vi "TxBfrPkt - Add Channels.vi"(6 "Ext Buffer?":bool, 7 "Add Port Channel?":bool, 8 "error in (no error)":errorcluster, 11 "Node Ptr":T1 format="%.0x") -> (0 "error out":errorcluster, 3 "Node Ptr out":T1 format="%.0x")   [LabVIEW 2016, in "UDP-Custom-Device System Explorer.lvlib"]
uses:
  UDP-Custom-Device System Explorer.lvlib
  <vilib>/NI Veristand/Custom Device API/Custom Device Item Ref.ctl
  <vilib>/NI Veristand/Custom Device API/Custom Device Channel.ctl
  <vilib>/NI Veristand/Custom Device API/Custom Device Channel Type.ctl
  <vilib>/NI VeriStand/Custom Device API/Custom Device API.lvlib
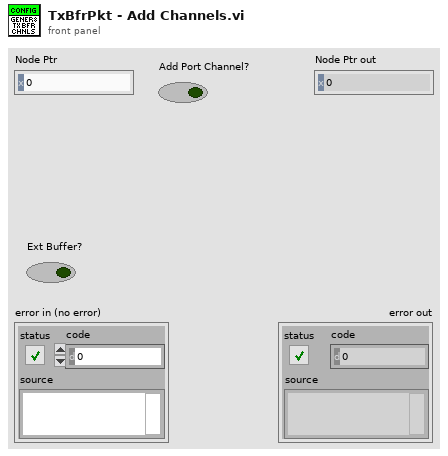
[diagram p1: front panel]
types:
  T1 = typedef "Custom Device API.lvlib/Custom Device Item Ref.ctl" = u64
  T2 = typedef "Custom Device API.lvlib/Custom Device Channel.ctl" = cluster{"Type":T3, "Units":string, "Default Value":dbl, "Faultable":bool, "Scalable":bool}
  T3 = typedef "Custom Device API.lvlib/Custom Device Channel Type.ctl" = enum16{"Input", "Output"}
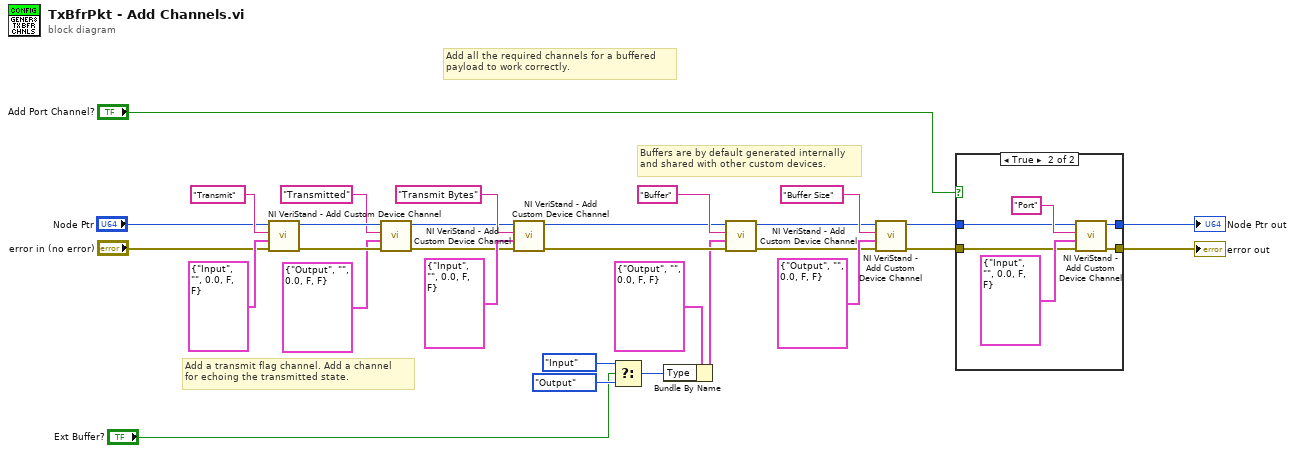
[diagram p0: block diagram]
diagram:
  # "Add a transmit flag channel. Add a channel\nfor echoing the transmitted state."
  # "Buffers are by default generated internally\nand shared with other custom devices."
  # "Add all the required channels for a buffered\npayload to work correctly."
  n1 = call <vilib>:"NI VeriStand - Add Custom Device Channel.vi"("error in (no error)"="error in (no error)", "Channel"=T2 {"Type"=enum."Input", "Units"="", "Default Value"=0.0, "Faultable"=FALSE, "Scalable"=FALSE}, "Channel Name"="Transmit", "Parent Ref in"="Node Ptr") -> ("error out"=w15:errorcluster, "Parent Ref out"=w17:T1)  [unwired: 4 in, 2 out]
  n2 = call <vilib>:"NI VeriStand - Add Custom Device Channel.vi"("error in (no error)"=w15, "Channel"=T2 {"Type"=enum."Output", "Units"="", "Default Value"=0.0, "Faultable"=FALSE, "Scalable"=FALSE}, "Channel Name"="Transmitted", "Parent Ref in"=w17) -> ("error out"=w14:errorcluster, "Parent Ref out"=w16:T1)  [unwired: 4 in, 2 out]
  n3 = call <vilib>:"NI VeriStand - Add Custom Device Channel.vi"("error in (no error)"=w14, "Channel"=T2 {"Type"=enum."Input", "Units"="", "Default Value"=0.0, "Faultable"=FALSE, "Scalable"=FALSE}, "Channel Name"="Transmit Bytes", "Parent Ref in"=w16) -> ("error out"=w24:errorcluster, "Parent Ref out"=w25:T1)  [unwired: 4 in, 2 out]
  n4 = Select(t=Custom_Device_Channel_Type."Input" ("Type"), s="Ext Buffer?", f=Custom_Device_Channel_Type."Output" ("Type")) -> (s? t:f=w21:T3)
  n5 = Bundle By Name(cluster=T2 {"Type"=enum."Output", "Units"="", "Default Value"=0.0, "Faultable"=FALSE, "Scalable"=FALSE} ("Channel"), "Type"=w21) -> (w18:T2)
  n6 = call <vilib>:"NI VeriStand - Add Custom Device Channel.vi"("error in (no error)"=w24, "Channel"=w18, "Channel Name"="Buffer", "Parent Ref in"=w25) -> ("error out"=w8:errorcluster, "Parent Ref out"=w9:T1)  [unwired: 4 in, 2 out]
  n7 = call <vilib>:"NI VeriStand - Add Custom Device Channel.vi"("error in (no error)"=w8, "Channel"=T2 {"Type"=enum."Output", "Units"="", "Default Value"=0.0, "Faultable"=FALSE, "Scalable"=FALSE}, "Channel Name"="Buffer Size", "Parent Ref in"=w9) -> ("error out"=w5:errorcluster, "Parent Ref out"=w3:T1)  [unwired: 4 in, 2 out]
  n8 = case shown="True" "Add Port Channel?" {
    tunnel: w5 -> [w31 w36]
    tunnel: w3 -> [w32 w35]
    tunnel: [w32 w34] -> w2
    tunnel: [w31 w33] -> w4
    frame False {
    }
    frame True {
      n9 = call <vilib>:"NI VeriStand - Add Custom Device Channel.vi"("error in (no error)"=w36, "Channel"=T2 {"Type"=enum."Input", "Units"="", "Default Value"=0.0, "Faultable"=FALSE, "Scalable"=FALSE}, "Channel Name"="Port", "Parent Ref in"=w35) -> ("error out"=w33:errorcluster, "Parent Ref out"=w34:T1)  [unwired: 4 in, 2 out]
    }
  }
  "error out" <- w4
  "Node Ptr out" <- w2
